vi "Set Output Mode.vi"(8 "error in (no error)":errorcluster caption="错误输入（无错误）", 10 "Output Mode":u32(ring) items=["Standby", "Operate"], 11 "5720A 输入":refnum<class "5720A.lvclass">) -> (0 "error out":errorcluster caption="错误输出", 3 "5720A 输出":refnum<class "5720A.lvclass">)   [LabVIEW 2020, in "5720A.lvlib" / "5720A.lvclass"]
uses:
  5720A.lvclass
  <instrlib>/Fluke 5XXX Series Multicalibrators/Fluke 5XXX Series Multicalibrators.lvlib
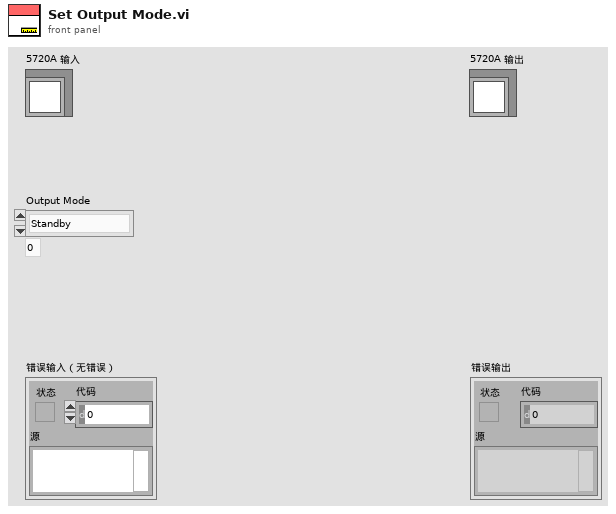
[diagram p1: front panel]
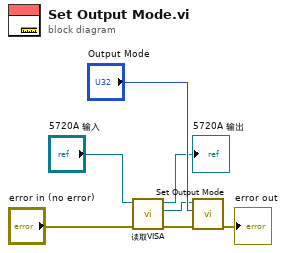
[diagram p0: block diagram]
diagram:
  n1 = call "读取VISA.vi"("error in (no error)"="error in (no error)", "多功能校准源接口输入"="5720A 输入") -> ("error out"=w2:errorcluster, "VISA"=w6:refnum<visa-resource-name>, "多功能校准源接口输出"=→"5720A 输出":refnum<class "5720A.lvclass">)  [unwired: 7 in]
  n2 = call <instrlib>:"Set Output Mode.vi"("error in (no error)"=w2, "Output Mode (0: Standby)"="Output Mode", "VISA resource name"=w6) -> ("error out"=→"error out":errorcluster)  [unwired: 7 in, 1 out]
